vi "SetUp.vi"(8 "error in (no error)":errorcluster, 11 "Prueba03 in":refnum<class "Prueba031.lvclass">) -> (0 "error out":errorcluster, 3 "Prueba03 out":refnum<class "Prueba031.lvclass">)   [LabVIEW 2019, in "Prueba031.lvclass"]
uses:
  Prueba031.lvclass
  Prueba031.lvclass/Prueba031.ctl
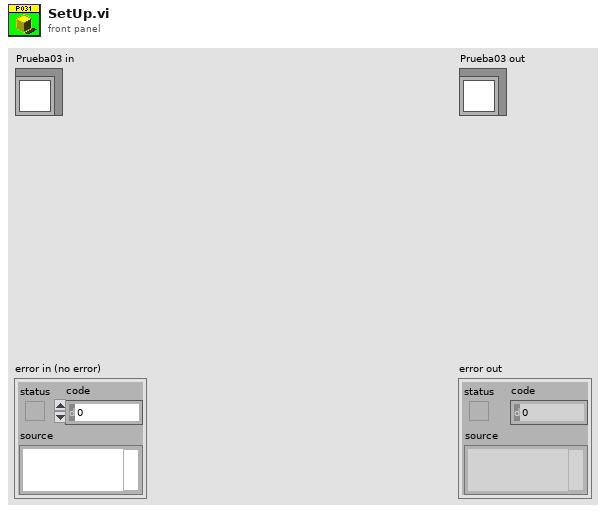
[diagram p1: front panel]
types:
  T1 = typedef "Prueba031.lvclass/BD.ctl" = cluster{"frec_referencia":dbl, "niv_presion_son_ref":dbl, "Incertidumbre":string[], "Tol +":string[], "Tol -":string[], "Referencia(dB)":string[], "Frecuencias(Hz)":string[], "vol_enviado_CAM":dbl, "CorreccionMic":string[]}
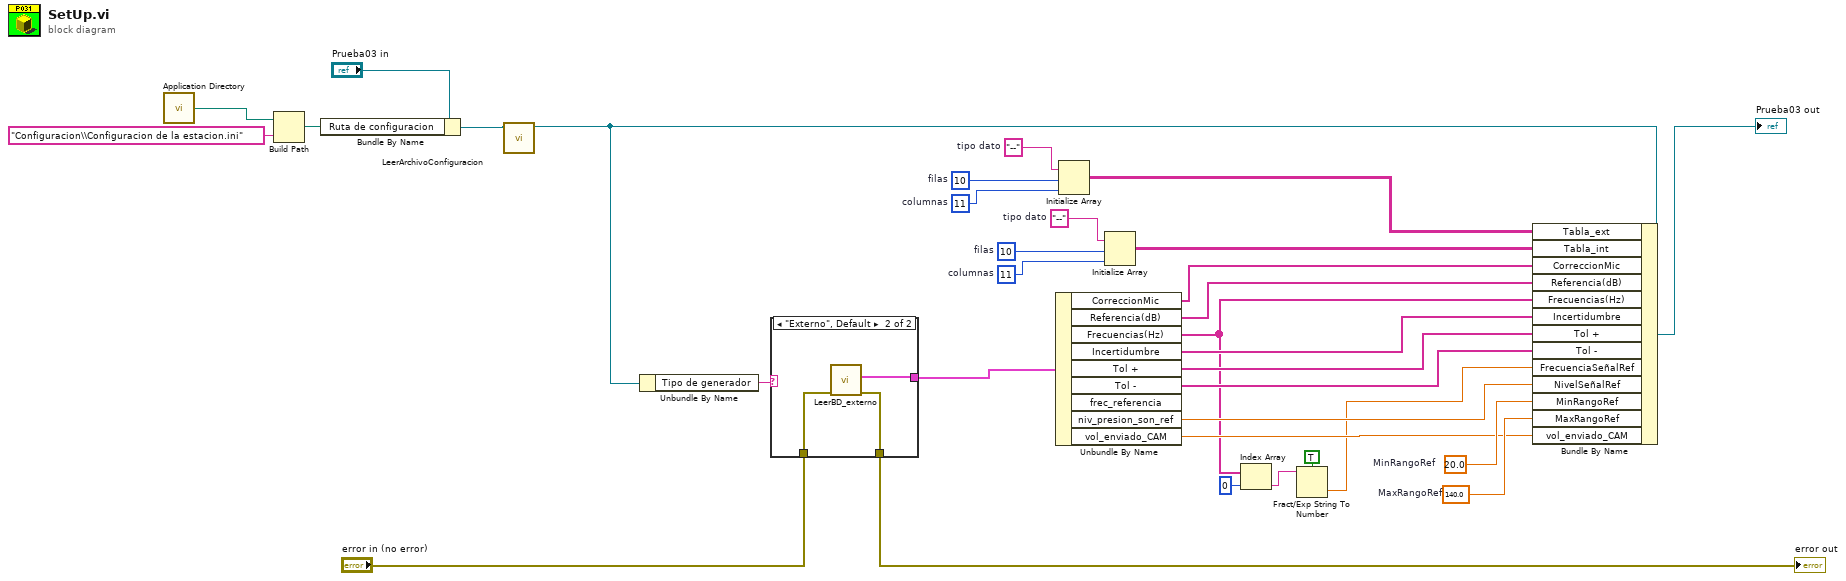
[diagram p0: block diagram]
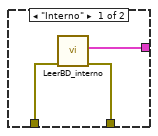
[diagram p2: hidden frame]
diagram:
  w16 = 11  # columnas
  w20 = 10  # filas
  w19 = "--"  # tipo dato
  w27 = 140.0  # MaxRangoRef
  w28 = 20.0  # MinRangoRef
  w31 = 11  # columnas
  w30 = 10  # filas
  w32 = "--"  # tipo dato
  n1 = call <vilib>:"Application Directory.vi"() -> ("Application Directory"=w13:path)
  n2 = Build Path(base path=w13, name or relative path="Configuracion\\Configuracion de la estacion.ini") -> (appended path=w12:path)
  n3 = Bundle By Name(cluster="Prueba03 in", "Ruta de configuracion"=w12) -> (w10:refnum<class "Prueba031.lvclass">)
  n4 = call "LeerArchivoConfiguracion.vi"("Prueba31 in"=w10) -> ("Prueba31 out"=w9:refnum<class "Prueba031.lvclass">)  [unwired: 9 in, 1 out]
  n5 = Unbundle By Name(w9) -> ("Tipo de generador"=w8:string)
  n6 = case shown="\"Externo\", Default" w8 {
    tunnel: "error in (no error)" -> [w36 w39]
    tunnel: [w35 w38] -> w26
    tunnel: [w34 w37] -> w25
    frame "Interno" {
      n7 = call "LeerBD_interno.vi"("error in (no error)"=w36) -> ("error out"=w35:errorcluster, "BD"=w34:T1)  [unwired: 8 in, 1 out]
    }
    frame "Externo", Default {
      n8 = call "LeerBD_externo.vi"("error in (no error)"=w39) -> ("error out"=w38:errorcluster, "BD"=w37:T1)  [unwired: 8 in, 1 out]
    }
  }
  "error out" <- w26
  n9 = Unbundle By Name(w25) -> ("CorreccionMic"=w6:string[], "Referencia(dB)"=w7:string[], "Frecuencias(Hz)"=w5:string[], "Incertidumbre"=w24:string[], "Tol +"=w23:string[], "Tol -"=w22:string[], "niv_presion_son_ref"=w21:dbl, "vol_enviado_CAM"=w15:dbl)  [unwired: 1 out]
  n10 = Initialize Array(w32, w30, w31) -> (w18:string[][])
  n11 = Initialize Array(w19, w20, w16) -> (w17:string[][])
  n12 = Index Array(array=w5, index=0) -> (element=w3:string)
  n13 = Fract/Exp String To Number(use system decimal point (T)=TRUE, string=w3) -> (number=w1:dbl)  [unwired: 2 in, 1 out]
  n14 = Bundle By Name(cluster=w9, "Tabla_ext"=w18, "Tabla_int"=w17, "CorreccionMic"=w6, "Referencia(dB)"=w7, "Frecuencias(Hz)"=w5, "Incertidumbre"=w24, "Tol +"=w23, "Tol -"=w22, "FrecuenciaSeñalRef"=w1, "NivelSeñalRef"=w21, "MinRangoRef"=w28, "MaxRangoRef"=w27, "vol_enviado_CAM"=w15) -> (→"Prueba03 out":refnum<class "Prueba031.lvclass">)
